vi "_FindPeakLocations.vi"(3 "threshold":dbl=100.0, 4 "Intensities":dbl[](array[numeric]), 5 "Masses":dbl[](array[numeric])) -> (0 "Peak List":T1[](array[typedef]), 2 "# found":i32)   [LabVIEW 2015]
uses:
  Type/_Peak Property.ctl
panel:
  out "Locations":dbl[](array[numeric])
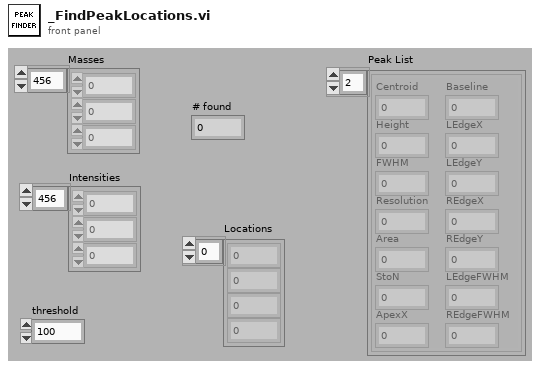
[diagram p1: front panel]
types:
  T1 = typedef "_Peak Property.ctl" = cluster{"Centroid":dbl, "Height":dbl, "FWHM":dbl, "Resolution":dbl, "Area":dbl, "StoN":dbl, "ApexX":dbl, "Baseline":dbl, "LEdgeX":dbl, "LEdgeY":dbl, "REdgeX":dbl, "REdgeY":dbl, "LEdgeFWHM":dbl, "REdgeFWHM":dbl}
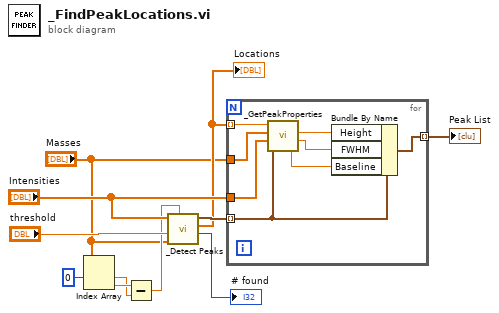
[diagram p0: block diagram]
diagram:
  n1 = Index Array(array="Masses", index #1=0 ("index")) -> (element #1=w4:dbl, element #2=w5:dbl)  [unwired: 1 in]
  n2 = Subtract(x=w5, y=w4) -> (x-y=w2:dbl)
  n3 = call "_Detect Peaks.vi"("X Step"=w2, "Masses"="Masses", "Minimum Height (0)"="threshold", "Original Data"="Intensities") -> ("# of Peaks"=→"# found":i32, "Locations"=w7:dbl[], "Peak List"=w9:T1[])  [unwired: 2 in]
  "Locations" <- w7
  n4 = for {
    tunnel: w7 -> [w17] mode=indexing
    tunnel: "Masses" -> [w19]
    tunnel: "Intensities" -> [w18]
    tunnel: [w15] -> w11 mode=indexing
    tunnel: w9 -> [w12] mode=indexing
    n5 = call "_GetPeakProperties.vi"("Peak"=w12, "Intensities"=w18, "Masses"=w19, "Location"=w17) -> ("Baseline"=w13:dbl, "FWHM"=w14:dbl, "Height"=w16:dbl)  [unwired: 1 out]
    n6 = Bundle By Name(cluster=w12, "Height"=w16, "FWHM"=w14, "Baseline"=w13) -> (w15:T1)
  }
  "Peak List" <- w11
